vi "shiftRegisterExample.vi"() -> ()   [LabVIEW 2014]
panel:
  out "All Result Array\nIndicator":dbl[](array[numeric])
  in  "Stop Value\nControl":dbl
  out "Result \nIndicator":dbl
  in  "Start Value\nControl":dbl
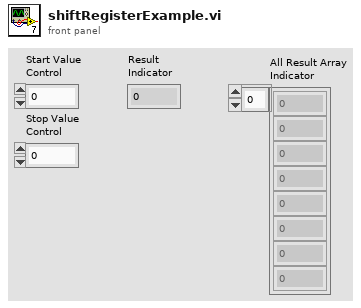
[diagram p1: front panel]
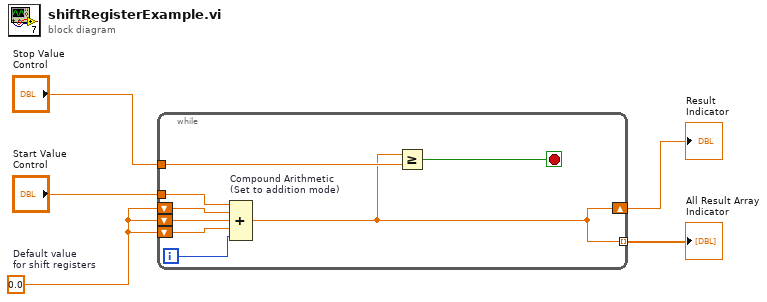
[diagram p0: block diagram]
diagram:
  w4 = 0.0  # Default value for shift registers
  n1 = while {
    tunnel: "Start Value\nControl" -> [w13]
    shift-right: [w7] -> w3
    shift-left: w4 -> [w12]
    shift-left: w4 -> [w11]
    shift-left: w4 -> [w10]
    tunnel: "Stop Value\nControl" -> [w9]
    tunnel: [w7] -> w1 mode=indexing
    i -> [w6]
    stop <- w8 stop-if-true
    n2 = Compound Arithmetic op=ADD "Compound Arithmetic\n(Set to addition mode)"(w13, w12, w11, w10, w6) -> (w7:dbl)
    n3 = Greater Or Equal?(x=w7, y=w9) -> (x >= y?=w8:bool)
  }
  "Result \nIndicator" <- w3
  "All Result Array\nIndicator" <- w1
